vi "calculate_Rgyro.vi"(1 "Previous Rest":dbl[](array[numeric]), 2 "angleYZ [rad]":dbl format="%#_13g", 3 "angleXZ [rad]":dbl format="%#_13g") -> (0 "Rgyro":dbl[](array[numeric]))   [LabVIEW 2015]
doc: "Calculates the Rgyro vector, which is necessary to perform further calculations in order to find the estimated gravity vector."
panel:
  out "RzGyro":dbl
  out "RyGyro":dbl
  out "RxGyro":dbl
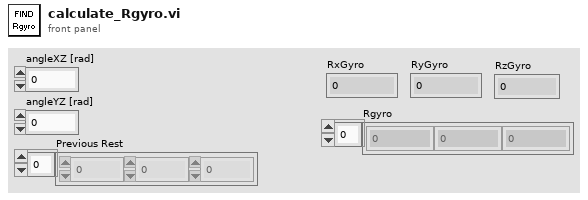
[diagram p1: front panel]
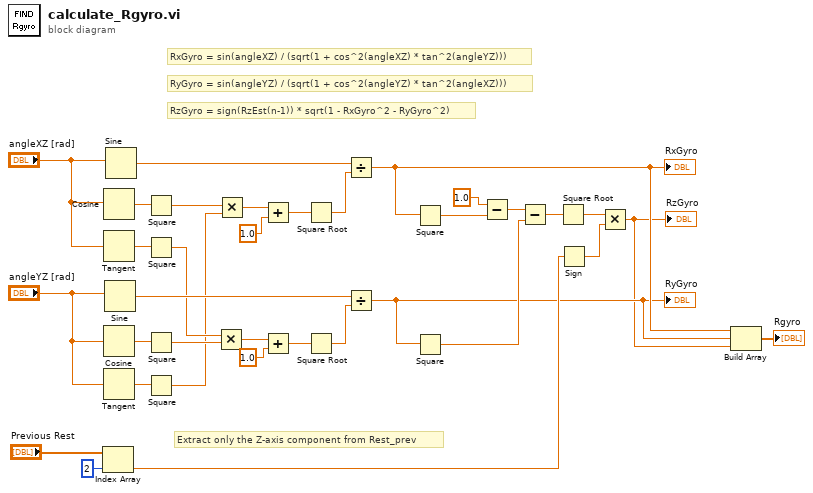
[diagram p0: block diagram]
diagram:
  # "Extract only the Z-axis component from Rest_prev"
  # "RzGyro = sign(RzEst(n-1)) * sqrt(1 - RxGyro^2 - RyGyro^2)"
  # "RyGyro = sin(angleYZ) / (sqrt(1 + cos^2(angleYZ) * tan^2(angleXZ)))"
  # "RxGyro = sin(angleXZ) / (sqrt(1 + cos^2(angleXZ) * tan^2(angleYZ)))"
  n1 = Index Array(array="Previous Rest", index=2) -> (element=w5:dbl)
  n2 = Cosine(x="angleXZ [rad]") -> (cos(x)=w32:dbl)
  n3 = Tangent(1:"angleXZ [rad]") -> (0:w31:dbl)
  n4 = Cosine(x="angleYZ [rad]") -> (cos(x)=w30:dbl)
  n5 = Tangent(1:"angleYZ [rad]") -> (0:w29:dbl)
  n6 = Sine(x="angleYZ [rad]") -> (sin(x)=w27:dbl)
  n7 = Sine(x="angleXZ [rad]") -> (sin(x)=w28:dbl)
  n8 = Square(x=w32) -> (x^2=w26:dbl)
  n9 = Square(x=w31) -> (x^2=w24:dbl)
  n10 = Square(x=w30) -> (x^2=w25:dbl)
  n11 = Square(x=w29) -> (x^2=w23:dbl)
  n12 = Multiply(x=w24, y=w25) -> (x*y=w21:dbl)
  n13 = Multiply(x=w26, y=w23) -> (x*y=w22:dbl)
  n14 = Add(x=w22, y=1.0) -> (x+y=w18:dbl)
  n15 = Add(x=w21, y=1.0) -> (x+y=w17:dbl)
  n16 = Square Root(x=w18) -> (sqrt(x)=w16:dbl)
  n17 = Square Root(x=w17) -> (sqrt(x)=w15:dbl)
  n18 = Divide(x=w28, y=w16) -> (x/y=w4:dbl)
  "RxGyro" <- w4
  n19 = Divide(x=w27, y=w15) -> (x/y=w3:dbl)
  "RyGyro" <- w3
  n20 = Square(x=w4) -> (x^2=w13:dbl)
  n21 = Square(x=w3) -> (x^2=w11:dbl)
  n22 = Subtract(x=1.0, y=w13) -> (x-y=w12:dbl)
  n23 = Subtract(x=w12, y=w11) -> (x-y=w10:dbl)
  n24 = Square Root(x=w10) -> (sqrt(x)=w9:dbl)
  n25 = Sign(1:w5) -> (0:w6:dbl)
  n26 = Multiply(x=w9, y=w6) -> (x*y=w2:dbl)
  "RzGyro" <- w2
  n27 = Build Array(w4, w3, w2) -> (→"Rgyro":dbl[])
